vi "Set_Window_Title.vi"(1 "Saved":bool, 2 "Current File":string, 3 "Application Name":string, 4 "VI Path":path) -> ()   [LabVIEW 2011]
doc: "This VI sets the title of a VI given by the \"VI Path\" parameter, in the format of \"Application Name: Current File *\", with the presence of \"*\" indicating that the \"Saved\" parameter is false."
panel:
  out "Application Name":string
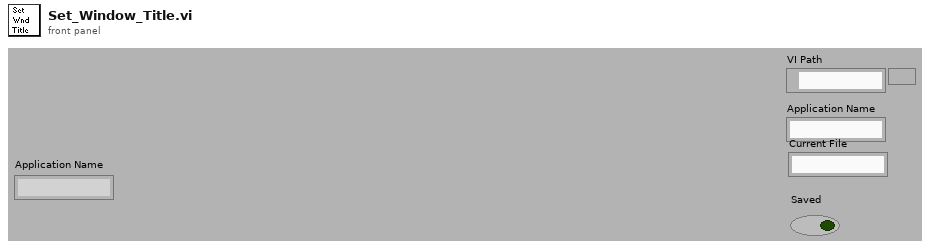
[diagram p1: front panel]
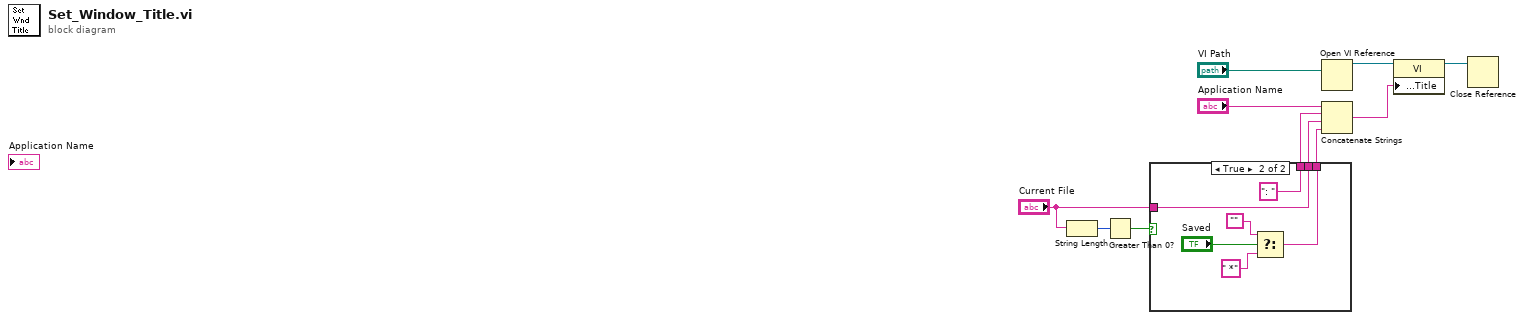
[diagram p0: block diagram]
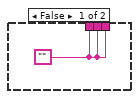
[diagram p2: hidden frame]
diagram:
  n1 = String Length(string="Current File") -> (length=w5:i32)
  n2 = Greater Than 0?(x=w5) -> (x > 0?=w2:bool)
  n3 = case shown="True" w2 {
    tunnel: [w12 w15] -> w7
    tunnel: [w12 w14] -> w4
    tunnel: "Current File" -> [_ w14]
    tunnel: [w12 ": " ("string")] -> w1
    frame False {
      w12 = ""
    }
    frame True {
      n4 = Select(t="", s="Saved", f=" *") -> (s? t:f=w15:string)
    }
  }
  n5 = Open VI Reference(vi path="VI Path") -> (vi reference=w11:refnum<vi>)  [unwired: 2 in, 4 out]
  n6 = Concatenate Strings("Application Name", w1, w4, w7) -> (w9:string)
  n7 = property class="VI"(reference=w11, "Front Panel.Title"=w9) -> (reference out=w10:refnum<vi>)  [unwired: 1 in, 1 out]
  n8 = Close Reference(reference=w10) -> ()  [unwired: 1 in, 1 out]
